vi "CH_LM Test Trigger.vi"() -> ()   [LabVIEW 2012, in "CH_LM.lvlib"]
doc: "This example VI starts the data acquisition and displays the measured data."
uses:
  CH_LM.lvlib
  CH_LM/CH_LM Measurement Delivery Mode.ctl
  CH_LM/CH_LM Streaming Data.ctl
  CH_LM/CH_LM Data Token.ctl
  CH_LM/CH_LM BaudRates.ctl
  CH_LM/CH_LM Parity.ctl
  CH_LM/CH_LM SerialConfiguration.ctl
  CH_LM/CH_LM Trigger Source.ctl
panel:
  out "Data Array size":i32
  out "Sequence ID":u32
  out "SID Missmatch":bool
  in  "Trigger Delay (0µs)":dbl format="%#.3g"
  in  "Trigger Slope (pos.)":bool=TRUE
  in  "Trigger Level (5%)":dbl=5.0 format="%#.3g"
  in  "Trigger Source":T1=enum."External"
  in  "Serial Configuration\n(19200,N,8,1)":T2={"Baud Rate"=19200, "Parity"=0, "Data Bits"=8, "Stop Bits"=1} {"Parity" items=["None", "Odd", "Even"]; "Baud Rate" items=["9600"=9600, "19200"=19200, "38400"=38400, "57600"=57600, "115200"=115200]}
  in  "Delivery Mode":T5=enum."Stream"
  in  "ID Query? (T: Yes)":bool
  in  "Reset? (F: No)":bool
  in  "Serial Number":string
  in  "Address":i32=1
  out "Data OK":bool
  out "Steaming Data Cluster":T6 {"Flags" format="%.0b"; "Unit ID" format="%.0b"; "Quad Distance"."Y" format="%#.1f"; "Quad Distance"."X" format="%#.1f"; "Value" format="%#.7e"}
  out "Data Header":bool
  in  "stopp":bool
  out "Data Tokens":T7[](array[typedef])=[enum."Raw data"]
  out "Stream error":errorcluster
  in  "Reset":bool
  out "Steaming Data Chart":cluster{"Value":sgl, u32, u32}[](graph)
  out "timed out?":bool
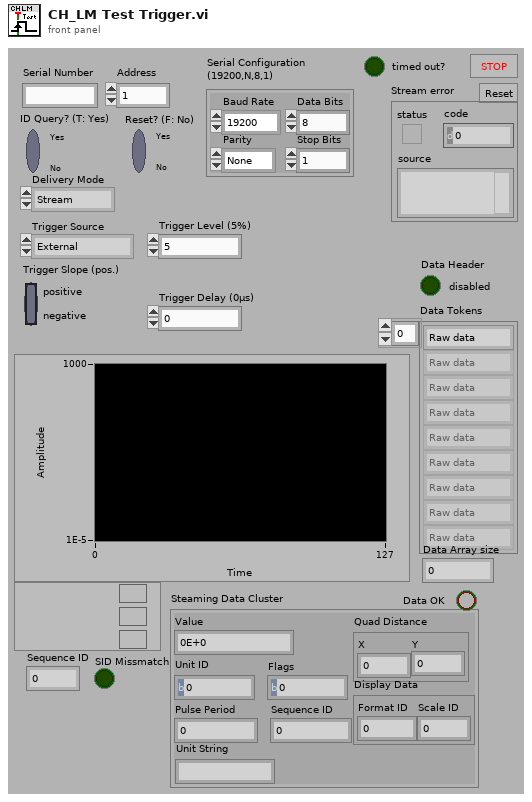
[diagram p1: front panel]
types:
  T1 = typedef "CH_LM.lvlib/CH_LM Trigger Source.ctl" = enum16{"Internal", "External", "Bus"}
  T2 = typedef "CH_LM.lvlib/CH_LM SerialConfiguration.ctl" = cluster{"Baud Rate":T3, "Parity":T4, "Data Bits":u16, "Stop Bits":u16}
  T3 = typedef "CH_LM.lvlib/CH_LM BaudRates.ctl" = u32
  T4 = typedef "CH_LM.lvlib/CH_LM Parity.ctl" = u16
  T5 = typedef "CH_LM.lvlib/CH_LM Measurement Delivery Mode.ctl" = enum16{"Last", "Stream"}
  T6 = typedef "CH_LM.lvlib/CH_LM Streaming Data.ctl" = cluster{"Value":sgl, "Quad Distance":cluster{"X":sgl, "Y":sgl}, "Display Data":cluster{"Format ID":u8, "Scale ID":u8}, "Unit ID":u8, "Flags":u32, "Pulse Period":u32, "Sequence ID":u32, "Unit String":string}
  T7 = typedef "CH_LM.lvlib/CH_LM Data Token.ctl" = enum16{"Raw data", "Quad distance", "Formated data", "Unit", "Pulse period", "Flags", "Sequence ID"}
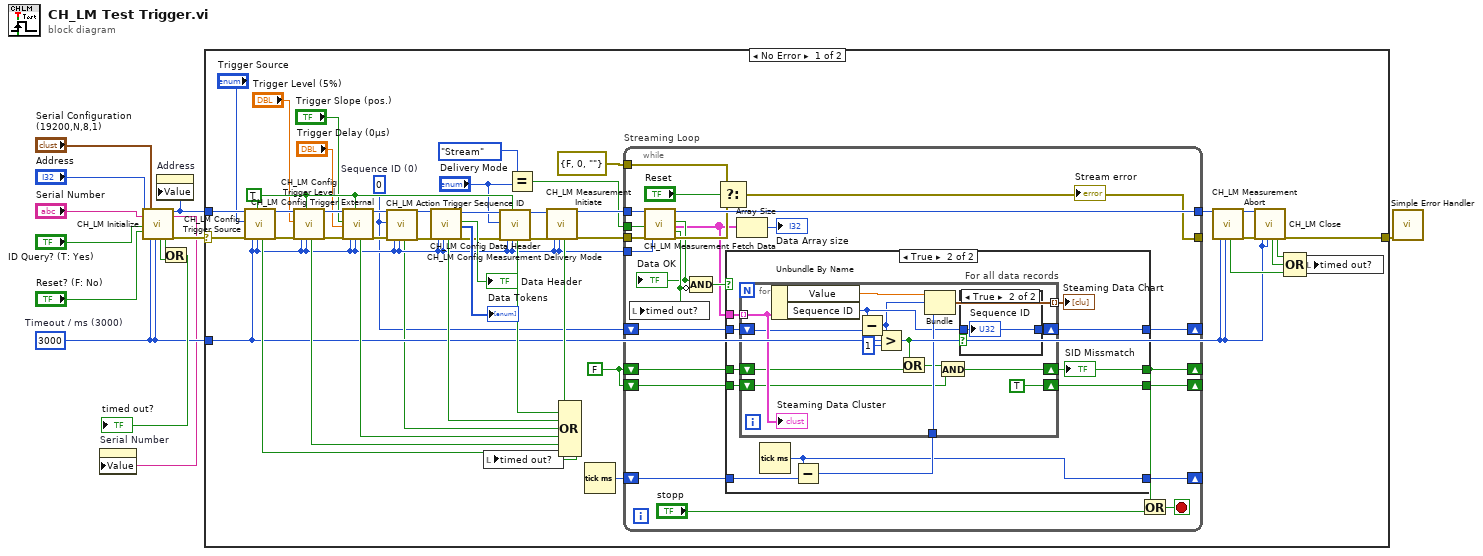
[diagram p0: block diagram]
diagram:
  w8 = 3000  # Timeout / ms (3000)
  n1 = call "CH_LM Initialize.vi"("Address"="Address", "Serial Number"="Serial Number", "ID Query (True)"="ID Query? (T: Yes)", "Reset (False)"="Reset? (F: No)", "Serial Configuration\n(19200,N,8,1)"="Serial Configuration\n(19200,N,8,1)", "Timeout / ms (3000)"=w8, "Lock Timeout / ms (1000)"=w8) -> ("Lock timed out"=w10:bool, "timed out?"=w11:bool, "Meter Index"=w2:i32, "Serial Number"=w1:string, "error out"=w7:errorcluster)  [unwired: 1 in, 7 out]
  n2 = property on="Serial Number" class="Str"("Value"=w1) -> ()  [unwired: 2 in, 2 out]
  n3 = property on="Address" class="DigNum (strict)"("Value"=w2) -> ()  [unwired: 2 in, 2 out]
  n4 = Or(x=w11, y=w10) -> (x .or. y?=→"timed out?":bool)
  n5 = case shown="No Error" w7 {
    selector: w7 -> [w37 w117]
    tunnel: w2 -> [w42 _]
    tunnel: w8 -> [w20 _]
    tunnel: [w43 w117] -> w4
    frame No Error {
      w17 = FALSE
      w18 = u32 0  # Sequence ID (0)
      w36 = TRUE ("Action (query)")
      n6 = call "CH_LM Config Trigger Source.vi"("Meter Index"=w42, "Trigger Source"="Trigger Source", "error in (no error)"=w37, "Timeout / ms (3000)"=w20, "Action (query)"=w36, "Lock Timeout / ms (1000)"=w20) -> ("Lock timed out"=w30:bool, "Meter Index"=w41:i32, "error out"=w38:errorcluster)  [unwired: 11 out]
      n7 = call "CH_LM Config Trigger Level.vi"("Meter Index"=w41, "Trigger Level (5%)"="Trigger Level (5%)", "error in (no error)"=w38, "Timeout / ms (3000)"=w20, "Action (query)"=w36, "Lock Timeout / ms (1000)"=w20) -> ("Lock timed out"=w31:bool, "Meter Index"=w40:i32, "error out"=w39:errorcluster)  [unwired: 11 out]
      n8 = call "CH_LM Config Trigger External.vi"("Meter Index"=w40, "Trigger Slope (pos.)"="Trigger Slope (pos.)", "Trigger Delay (0µs)"="Trigger Delay (0µs)", "error in (no error)"=w39, "Timeout / ms (3000)"=w20, "Action (query)"=w36, "Lock Timeout / ms (1000)"=w20) -> ("Lock timed out"=w32:bool, "Meter Index"=w24:i32, "error out"=w23:errorcluster)  [unwired: 10 out]
      n9 = call "CH_LM Action Trigger Sequence ID.vi"("Meter Index"=w24, "Sequence ID (0)"=w18, "error in (no error)"=w23, "Timeout / ms (3000)"=w20, "Lock Timeout / ms (1000)"=w20) -> ("Lock timed out"=w19:bool, "Meter Index"=w21:i32, "error out"=w22:errorcluster)  [unwired: 12 out]
      n10 = call "CH_LM Config Data Header.vi"("Meter Index"=w21, "error in (no error)"=w22, "Timeout / ms (3000)"=w20, "Lock Timeout / ms (1000)"=w20) -> ("Lock timed out"=w33:bool, "Meter Index"=w46:i32, "Data Header"=→"Data Header":bool, "Data Tokens"=→"Data Tokens":T7[], "error out"=w45:errorcluster)  [unwired: 3 in, 8 out]
      n11 = call "CH_LM Config Measurement Delivery Mode.vi"("Meter Index"=w46, "Delivery Mode"="Delivery Mode", "error in (no error)"=w45, "Timeout / ms (3000)"=w20, "Action (query)"=w36, "Lock Timeout / ms (1000)"=w20) -> ("Lock timed out"=w34:bool, "Meter Index"=w47:i32, "error out"=w44:errorcluster)  [unwired: 11 out]
      n12 = Equal?(x=CH_LM_Measurement_Delivery_Mode."Stream" ("Delivery Mode"), y="Delivery Mode") -> (x = y?=w14:bool)
      n13 = call "CH_LM Measurement Initiate.vi"("Meter Index"=w47, "error in (no error)"=w44, "Timeout / ms (3000)"=w20, "Lock Timeout / ms (1000)"=w20) -> ("Lock timed out"=w35:bool, "Meter Index"=w58:i32, "error out"=w56:errorcluster)  [unwired: 13 out]
      n14 = Compound Arithmetic op=OR(w35, w34, w33, w19, w32, w31, w30) -> (w29:bool)
      n15 = local write "timed out?"(w29) -> ()
      n16 = Tick Count (ms)() -> (millisecond timer value=w54:u32)
      n17 = while "Streaming Loop" {
        tunnel: w58 -> [w84]
        tunnel: [w83] -> w57
        tunnel: w20 -> [w82]
        tunnel: errorcluster {"status"=FALSE, "code"=0, "source"=""} ("error in (no error)") -> [w80]
        shift-right: [w77] -> _
        shift-left: w54 -> [w78]
        shift-right: [w71] -> _
        shift-left: w18 -> [w70]
        shift-right: [w64] -> _
        shift-left: w17 -> [w69]
        shift-right: [w67] -> _
        shift-left: w17 -> [w68]
        tunnel: w14 -> [w63]
        tunnel: w56 -> [w75]
        tunnel: [w76] -> _
        stop <- w65 stop-if-true
        n18 = call "CH_LM Measurement Fetch Data.vi"("Meter Index"=w84, "All Records? (F)"=w63, "error in (no error)"=w75, "Timeout / ms (1000)"=w82) -> ("Meter Index"=w83:i32, "Data OK"=w73:bool, "Data Array"=w62:T6[], "timed out?"=w74:bool, "error out"=w79:errorcluster)  [unwired: 1 in, 10 out]
        "Data OK" <- w73
        n19 = local write "timed out?"(w74) -> ()
        n20 = Compound Arithmetic op=AND(w73, invert w74) -> (w72:bool)
        n21 = Select(t=w80, s="Reset", f=w79) -> (s? t:f=w76:errorcluster)
        "Stream error" <- w76
        n22 = case shown="True" w72 {
          tunnel: w62 -> [_ w99]
          tunnel: w78 -> [w88 w98]
          tunnel: [w88 w96] -> w77
          tunnel: [w87 w94] -> w71
          tunnel: w70 -> [w87 w93]
          tunnel: w69 -> [w86 w92]
          tunnel: [w86 w89] -> w64
          tunnel: w68 -> [w85 w91]
          tunnel: [w85 w90] -> w67
          frame False {
          }
          frame True {
            n23 = Tick Count (ms)() -> (millisecond timer value=w96:u32)
            n24 = Subtract(x=w96, y=w98) -> (x-y=w97:u32)
            n25 = for "For all data records" {
              tunnel: w99 -> [w114] mode=indexing
              tunnel: [w112] -> w95 mode=indexing
              tunnel: w97 -> [w111]
              shift-right: [w100] -> w94
              shift-left: w93 -> [w109]
              shift-right: [w104] -> w89
              shift-left: w92 -> [w108]
              shift-right: [TRUE] -> w90
              shift-left: w91 -> [w103]
              n26 = Unbundle By Name(w114) -> ("Value"=w113:sgl, "Sequence ID"=w110:u32)
              n27 = Subtract(x=w110, y=w109) -> (x-y=w107:u32)
              n28 = Greater?(x=w107, y=u32 1) -> (0:w101:bool)
              n29 = Or(x=w101, y=w108) -> (x .or. y?=w105:bool)
              n30 = Bundle("Value"=w113, w107, w111) -> (w112:cluster{"Value":sgl, u32, u32})  [unwired: 1 out]
              n31 = And(x=w105, y=w103) -> (x .and. y?=w104:bool)
              n32 = case shown="True" w101 {
                tunnel: w110 -> [w115 w116]
                tunnel: [w115 w116] -> w100
                frame False {
                }
                frame True {
                  "Sequence ID" <- w116
                }
              }
              "Steaming Data Cluster" <- w114
            }
            "Steaming Data Chart" <- w95
            "SID Missmatch" <- w89
          }
        }
        n33 = Array Size(array=w62) -> (size(s)=→"Data Array size":i32)
        n34 = Or(x=w64, y="stopp") -> (x .or. y?=w65:bool)
      }
      n35 = call "CH_LM Measurement Abort.vi"("Meter Index"=w57, "Timeout / ms (3000)"=w20, "Lock Timeout / ms (1000)"=w20) -> ("Lock timed out"=w51:bool, "Meter Index"=w59:i32, "error out"=w60:errorcluster)  [unwired: 1 in, 13 out]
      n36 = call "CH_LM Close.vi"("Meter Index"=w59, "error in (no error)"=w60, "Timeout / ms (3000)"=w20, "Lock Timeout / ms (1000)"=w20) -> ("Lock timed out"=w49:bool, "timed out?"=w50:bool, "error out"=w43:errorcluster)  [unwired: 13 out]
      n37 = Compound Arithmetic op=OR(w50, w49, w51) -> (w48:bool)
      n38 = local write "timed out?"(w48) -> ()
    }
    frame Error {
    }
  }
  n39 = call <vilib>:"Simple Error Handler.vi"("error in (no error)"=w4) -> ()  [unwired: 1 in, 8 out]
